vi "Del.vi"(0 "reference in":refnum<class "Redis.lvclass">, 1 "Keys":string[](array[string]), 11 "Error In":errorcluster) -> (4 "reference out":refnum<class "Redis.lvclass">, 8 "Length":i64, 15 "Error Out":errorcluster)   [LabVIEW 2020, in "Redis.lvclass"]
doc: "<b>DEL</b>\n\nRemoves the specified keys. A key is ignored if it does not exist."
uses:
  Redis.lvclass
  Redis.lvclass/Redis.ctl
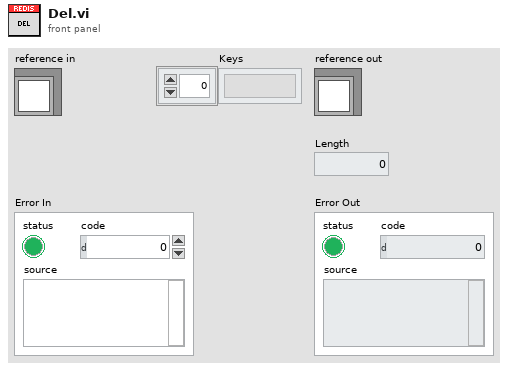
[diagram p1: front panel]
types:
  T1 = typedef "Redis.lvclass/RedisDataType.ctl" = cluster{"Reply Type":T2, "Integer":i64, "String":string, "Multibulk":variant[], "StringData":string[]}
  T2 = typedef "Redis.lvclass/ReplyDataTypeEnum.ctl" = enum16{"None", "Error", "Status", "Nil", "Integer", "String", "Multibulk"}
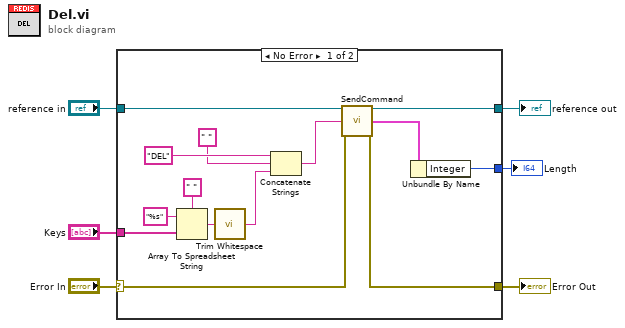
[diagram p0: block diagram]
diagram:
  n1 = case shown="No Error" "Error In" {
    selector: "Error In" -> [w18 w22]
    tunnel: [w17 w22] -> w5
    tunnel: [w20 w21] -> w3
    tunnel: "reference in" -> [w19 w21]
    tunnel: "Keys" -> [w7 _]
    tunnel: [w12 _] -> w1
    frame No Error {
      n2 = Array To Spreadsheet String(delimiter (Tab)=" ", array=w7, 3:"%s" ("format string")) -> (spreadsheet string=w11:string)
      n3 = call <vilib>:"Trim Whitespace.vi"("string"=w11) -> ("trimmed string"=w8:string)  [unwired: 1 in]
      n4 = Concatenate Strings("DEL", " ", w8) -> (w15:string)
      n5 = call "SendCommand.vi"("reference in"=w19, "Command"=w15, "Error In"=w18) -> ("reference out"=w20:refnum<class "Redis.lvclass">, "Data"=w13:T1, "Error Out"=w17:errorcluster)  [unwired: 10 in]
      n6 = Unbundle By Name(w13) -> ("Integer"=w12:i64)
    }
    frame Error {
    }
  }
  "Error Out" <- w5
  "reference out" <- w3
  "Length" <- w1
